vi "Config.vi"(0 "class data in":refnum<class "AnalogComparator.lvclass">, 5 "SettinganalogComp":T1) -> (4 "class data out":refnum<class "AnalogComparator.lvclass">)   [LabVIEW 2019, in "AnalogComparator.lvclass"]
uses:
  AnalogComparator.lvclass
  TypeDef/ConfigAnalogComp.ctl
  AnalogComparator.lvclass/AnalogComparator.ctl
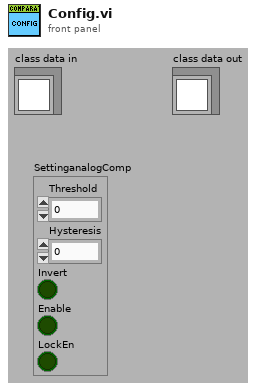
[diagram p1: front panel]
types:
  T1 = typedef "ConfigAnalogComp.ctl" = cluster{"Threshold":dbl, "Hysteresis":dbl, "Invert":bool, "Enable":bool, "LockEn":bool}
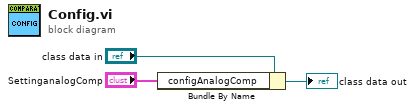
[diagram p0: block diagram]
diagram:
  n1 = Bundle By Name(cluster="class data in", "configAnalogComp"="SettinganalogComp") -> (→"class data out":refnum<class "AnalogComparator.lvclass">)
